vi "UTL_EraseGlobals.vi"(8 "error in (no error)":errorcluster) -> (0 "error out":errorcluster)   [LabVIEW 2019]
uses:
  Variable global de carga.vi
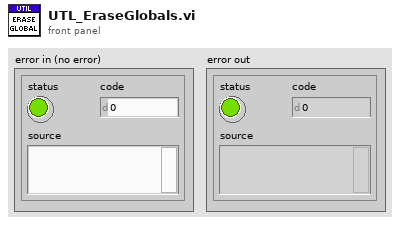
[diagram p1: front panel]
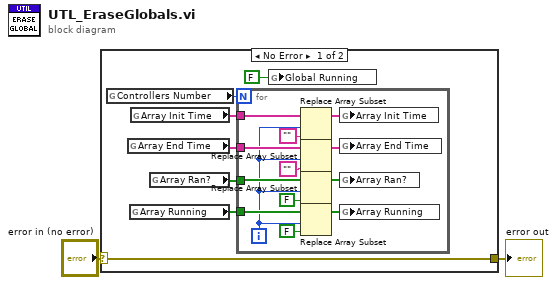
[diagram p0: block diagram]
diagram:
  n1 = case shown="No Error" "error in (no error)" {
    selector: "error in (no error)" -> [w9 w23]
    tunnel: [w9 w23] -> w1
    frame No Error {
      n2 = global read "Variable global de carga.vi" "Controllers Number"() -> (w3:u16)
      n3 = global read "Variable global de carga.vi" "Array End Time"() -> (w6:string[])
      n4 = global read "Variable global de carga.vi" "Array Running"() -> (w4:bool[])
      n5 = global read "Variable global de carga.vi" "Array Init Time"() -> (w7:string[])
      n6 = global read "Variable global de carga.vi" "Array Ran?"() -> (w5:bool[])
      n7 = for {
        N: w3 -> [_]
        tunnel: w7 -> [w21]
        tunnel: w6 -> [w19]
        tunnel: w5 -> [w18]
        tunnel: w4 -> [w15]
        i -> [w14]
        n8 = Replace Array Subset(array=w21, new element="", index=w14) -> (w13:string[])
        n9 = Replace Array Subset(array=w19, new element="", index=w14) -> (w10:string[])
        n10 = Replace Array Subset(array=w18, new element=FALSE ("new element/subarray"), index=w14) -> (w11:bool[])
        n11 = Replace Array Subset(array=w15, new element=FALSE ("new element/subarray"), index=w14) -> (w12:bool[])
        n12 = global write "Variable global de carga.vi" "Array Init Time"(w13) -> ()
        n13 = global write "Variable global de carga.vi" "Array End Time"(w10) -> ()
        n14 = global write "Variable global de carga.vi" "Array Ran?"(w11) -> ()
        n15 = global write "Variable global de carga.vi" "Array Running"(w12) -> ()
      }
      n16 = global write "Variable global de carga.vi" "Global Running"(FALSE ("Global Running")) -> ()
    }
    frame Error {
    }
  }
  "error out" <- w1
